vi "Stop Move piezo.vi"(8 "error in (no error)":errorcluster, 10 "MOVE TO [MICRON]":dbl=1.0 format="%0.2f", 11 "Cluster 2":T1={"serial number"="Dev5/ao0", "handle"=10, "status"=0, "range"=0}) -> (0 "error out":errorcluster)   [LabVIEW 2013, in "Piezo.lvlib"]
uses:
  Piezo/Piezo.lvlib
  Hardware Configuration Piezo NEW.ctl
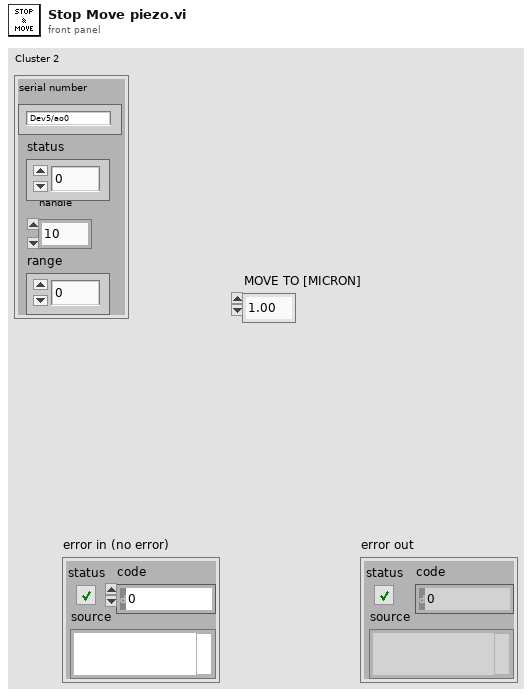
[diagram p1: front panel]
types:
  T1 = typedef "Hardware Configuration Piezo NEW.ctl" = cluster{"serial number":string, "handle":i32, "status":i32, "range":i32}
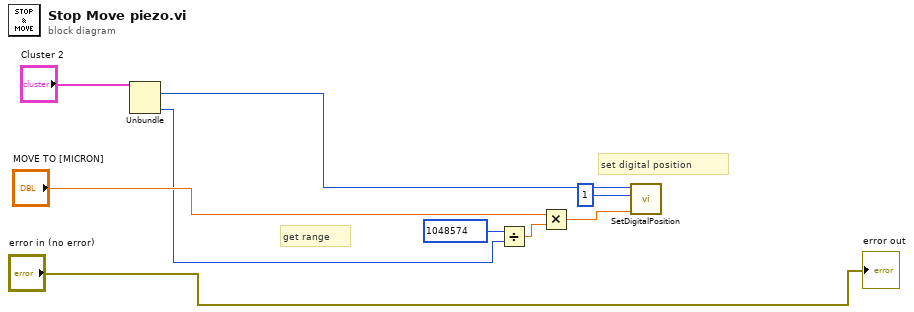
[diagram p0: block diagram]
diagram:
  # "get range"
  # "set digital position"
  n1 = Unbundle("Cluster 2") -> ("handle"=w8:i32, "range"=w5:i32)  [unwired: 2 out]
  n2 = Divide(x=1048574, y=w5) -> (x/y=w2:dbl)
  n3 = Multiply(x="MOVE TO [MICRON]", y=w2) -> (x*y=w1:dbl)
  n4 = call "SetDigitalPosition.vi"("Position"=w1, "Controller Channel"=1, "Handle"=w8) -> ()  [unwired: 8 in, 1 out]
  "error out" <- "error in (no error)"
